vi "Do Request.vi"(7 "Processing In":refnum<class "Processing.lvclass">, 11 "HomeHTTPController in":refnum<class "HomeHTTPController.lvclass">) -> (0 "error out":errorcluster, 5 "Processing":refnum<class "Processing.lvclass">)   [LabVIEW 2020, in "Volatus.lvlib" / "HomeHTTPController.lvclass"]
doc: "A controller's main job is to respond to a request by generating a response. The response value must be specified by calling Set Response.vi on the Processing class that's passed through the VI otherwise an error will be generated.\n\nThere are several helpers available for common response types:\nGenerating HTML content programmatically - Create Basic Response.vi\nStreaming a file from disk - Create File Response.vi\nRedirecting the user to another URL - Create Redirect Response.vi\n\nFile responses are streamed in chunks and do not load the entire file into memory at once to send in the response which allows serving large files more efficiently."
uses:
  HomeHTTPController.lvclass
  HomeHTTPController.lvclass/HomeHTTPController.ctl
  lv-http-server/HTTP Server/Processing/Processing.lvclass
  lv-http-util/HTTP Utils/Response/Response.lvclass
  VolatusApiHttpService/VolatusApiHttpService.lvclass
  C:/dev/lv20CE/relink/lv-volatus/Volatus/VolatusApiHttpService/VolatusApiHttpService.lvclass
  C:/dev/lv20CE/relink/lv-http-server/HTTP Server/Service/Service.lvclass
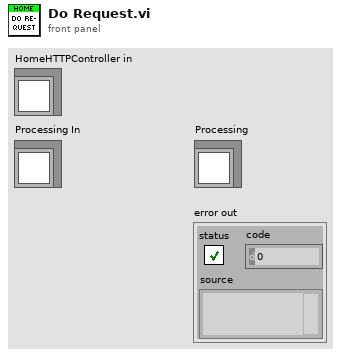
[diagram p1: front panel]
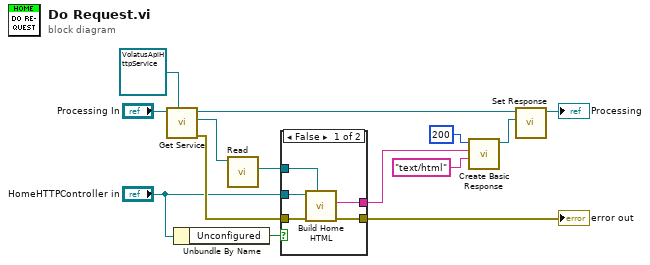
[diagram p0: block diagram]
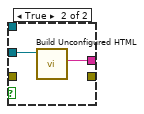
[diagram p2: hidden frame]
diagram:
  n1 = call "Get Service.vi"("Service Type"=refnum<class "VolatusApiHttpService.lvclass"> refnum ("Volatus:VolatusApiHttpService.lvclass"), "Processing in"="Processing In") -> ("error out"=w14:errorcluster, "Service"=w3:refnum<class "VolatusApiHttpService.lvclass">, "Processing out"=w5:refnum<class "Processing.lvclass">)  [unwired: 7 in]
  n2 = Unbundle By Name("HomeHTTPController in") -> ("Unconfigured"=w7:bool)
  n3 = call "Read.vi"("VolatusApiHttpService in"=w3) -> ("VolatusAPI"=w1:refnum<class "VolatusAPI.lvclass">)  [unwired: 10 in]
  n4 = case shown="False" w7 {
    tunnel: "HomeHTTPController in" -> [w19 w21]
    tunnel: [w18 w20] -> w6
    tunnel: w1 -> [w17 _]
    tunnel: w14 -> [w16 _]
    tunnel: [w15 _] -> w2
    frame False {
      n5 = call "Build Home HTML.vi"("Volatus:VolatusAPI"=w17, "error in (no error)"=w16, "HomeHTTPController in"=w19) -> ("error out"=w15:errorcluster, "Home HTML"=w18:string)  [unwired: 6 in, 1 out]
    }
    frame True {
      n6 = call "Build Unconfigured HTML.vi"("HomeHTTPController in"=w21) -> ("Unconfigured HTML"=w20:string)  [unwired: 8 in, 2 out]
    }
  }
  "error out" <- w2
  n7 = call "Create Basic Response.vi"("Content-Type (text/plain)"="text/html", "Payload"=w6, "Status Code"=u16 200) -> ("Response out"=w12:refnum<class "Response.lvclass">)  [unwired: 7 in, 1 out]
  n8 = call "Set Response.vi"("Response"=w12, "Processing in"=w5) -> ("Processing out"=→"Processing":refnum<class "Processing.lvclass">)  [unwired: 9 in]
